vi "Increment_Cost_Function_for_Jumps(11)-1.vi"(1 "[IN] Subtrack":T1) -> (0 "[OUT] Subtrack":T1)   [LabVIEW 2013]
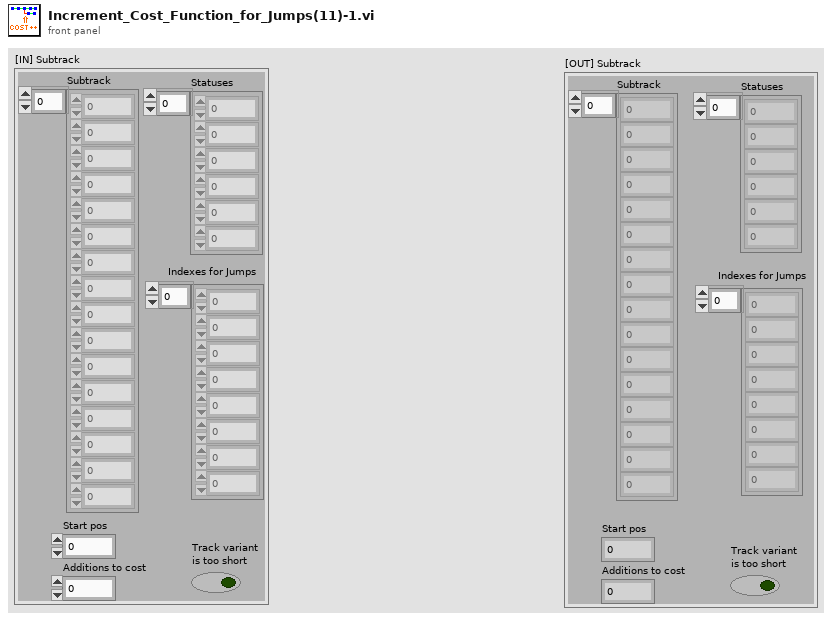
[diagram p1: front panel]
types:
  T1 = cluster{"Subtrack":dbl[], "Statuses":i16[], "Start pos":i32, "Additions to cost":i32, "Track variant \nis too short":bool, "Indexes for Jumps":i32[]}
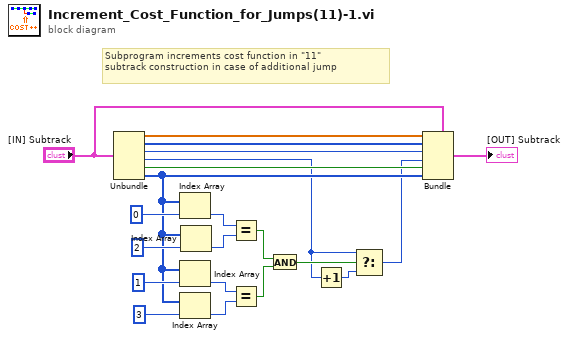
[diagram p0: block diagram]
diagram:
  # "Subprogram increments cost function in \"11\" \nsubtrack construction in case of additional jump"
  n1 = Unbundle("[IN] Subtrack") -> ("Subtrack"=w20:dbl[], "Statuses"=w21:i16[], "Start pos"=w19:i32, "Additions to cost"=w3:i32, "Track variant \nis too short"=w16:bool, "Indexes for Jumps"=w9:i32[])
  n2 = Index Array(array=w9, index=0) -> (element=w13:i32)
  n3 = Index Array(array=w9, index=1) -> (element=w8:i32)
  n4 = Index Array(array=w9, index=3) -> (element=w7:i32)
  n5 = Index Array(array=w9, index=2) -> (element=w12:i32)
  n6 = Equal?(x=w13, y=w12) -> (x = y?=w6:bool)
  n7 = Equal?(x=w8, y=w7) -> (x = y?=w5:bool)
  n8 = And(x=w6, y=w5) -> (x .and. y?=w4:bool)
  n9 = Increment(x=w3) -> (x+1=w2:i32)
  n10 = Select(t=w3, s=w4, f=w2) -> (s? t:f=w1:i32)
  n11 = Bundle(cluster="[IN] Subtrack", "Subtrack"=w20, "Statuses"=w21, "Start pos"=w19, "Additions to cost"=w1, "Track variant \nis too short"=w16, "Indexes for Jumps"=w9) -> (→"[OUT] Subtrack":T1)
